vi "De-Commentify.vi"(2 "Comment Token":string, 3 "File Text":string) -> (0 "Comments Out":string[](array[string]), 1 "Text Out":string)   [LabVIEW 2016]
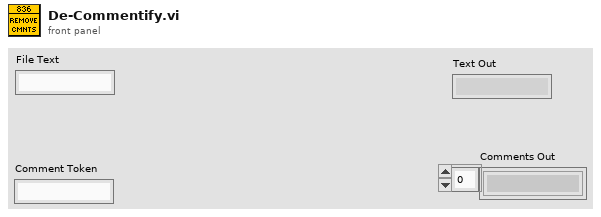
[diagram p1: front panel]
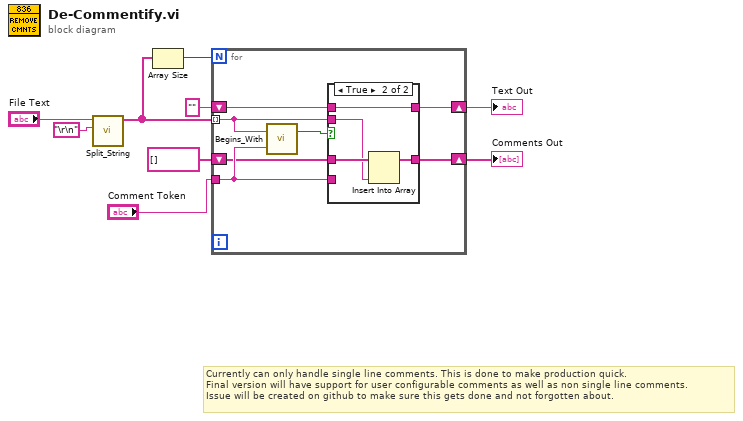
[diagram p0: block diagram]
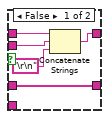
[diagram p2: hidden frame]
diagram:
  # "Currently can only handle single line comments. This is done to make production quick.\nFinal version will have support for user configurable comments as well as non single line comments.\nIssue will be created on github to make sure this gets done and not forgotten about."
  n1 = call <userlib>:"Split_String.vi"("Delim Char"="\r\n", "Text In"="File Text") -> ("Splits Out"=w5:string[])  [unwired: 8 in, 1 out]
  n2 = Array Size(array=w5) -> (size(s)=w7:i32)
  n3 = for {
    N: w7 -> [_]
    tunnel: "Comment Token" -> [w12]
    tunnel: w5 -> [w15] mode=indexing
    shift-right: [w13] -> w3
    shift-left: "" -> [w14]
    shift-right: [w10] -> w1
    shift-left: string[] [] -> [w11]
    n4 = call <userlib>:"Begins_With.vi"("Beginning"=w12, "String"=w15) -> ("Begins With?"=w16:bool)  [unwired: 1 out]
    n5 = case shown="True" w16 {
      tunnel: w15 -> [w19 w22]
      tunnel: w14 -> [w21 w25]
      tunnel: [w20 w25] -> w13
      tunnel: w12 -> [_ _]
      tunnel: w11 -> [w18 w24]
      tunnel: [w18 w23] -> w10
      frame False {
        n6 = Concatenate Strings(w21, w19, "\r\n") -> (w20:string)
      }
      frame True {
        n7 = Insert Into Array(array=w24, new element=w22) -> (w23:string[])  [unwired: 1 in]
      }
    }
  }
  "Text Out" <- w3
  "Comments Out" <- w1
